vi "flattenTemperatureAbsToXML.vi"   [LabVIEW 2012, in "UnitsAndXML.lvlib"]
doc: "Generates an XML string for <B>temperatureAbs</B> in the unit specified in <B>temperatureAbsUnitInXML</B>. Connect <B>temperatureAbs</B> and <B>temperatureAbsAgain</B> to the same source. The VI uses <B>temperatureAbsAgain</B> to obtain the data name."
uses:
  <userlib>/Common/UnitsAndXML/UnitsAndXML.lvlib
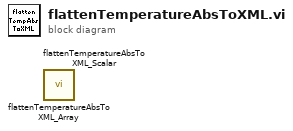
[diagram p0: block diagram]
diagram:
  n1 = call <userlib>:"flattenTemperatureAbsToXML_Array.vi"() -> ()  [unwired: 10 in, 2 out]
  n2 = call <userlib>:"flattenTemperatureAbsToXML_Scalar.vi"() -> ()  [unwired: 10 in, 2 out]
